vi "Load XML.vi"() -> (3 "Map":map{string, T1}(c390))   [LabVIEW 2021]
uses:
  bd.ctl
  Node/Node.lvclass
  wire.ctl
  <vilib>/xml/Load XML File.vi
  <vilib>/xml/NI_XML.lvlib
  <vilib>/httpClient/LabVIEWHTTPClient.lvlib
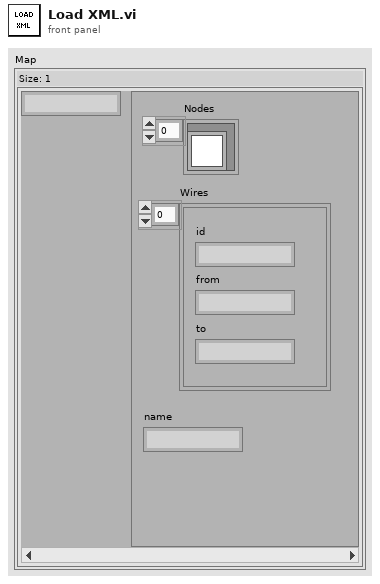
[diagram p1: front panel]
types:
  T1 = typedef "bd.ctl" = cluster{"Nodes":refnum<class "Node.lvclass">[], "Wires":T2[], "name":string}
  T2 = typedef "wire.ctl" = cluster{"id":string, "from":string, "to":string}
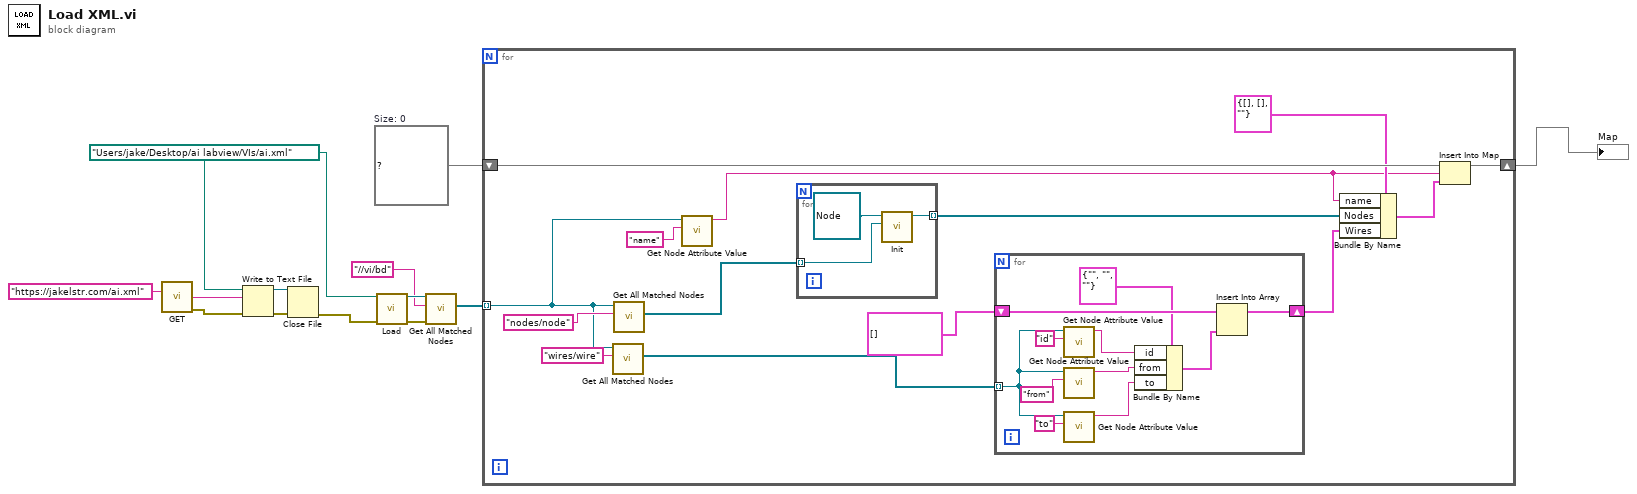
[diagram p0: block diagram]
diagram:
  w10 = map{string, T1} {}  # Size: 0
  w1 = path "/Users/jake/Desktop/ai labview/VIs/ai.xml" ("path to XML document")
  n1 = call <vilib>:"GET.vi"("url"="https://jakelstr.com/ai.xml") -> ("body"=w5:string, "error out"=w6:errorcluster)  [unwired: 11 in, 2 out]
  n2 = Write to Text File(file (use dialog)=w1, text=w5, error in=w6) -> (refnum out=w3:refnum<file>, error out=w4:errorcluster)  [unwired: 1 in, 1 out]
  n3 = Close File(refnum=w3, error in=w4) -> (error out=w2:errorcluster)  [unwired: 1 out]
  n4 = call-poly <vilib>:"Load.vi"("path to XML document"=w1, "error in (no error)"=w2) -> ("DOM document out"=w12:refnum<k20>, "error out"=w13:errorcluster)  [unwired: 11 in, 1 out]
  n5 = call <vilib>:"Get All Matched Nodes.vi"("error in (no error)"=w13, "XPath expression"="//vi/bd", "node in"=w12) -> ("node result array"=w9:refnum<k20>[])  [unwired: 6 in, 2 out]
  n6 = for {
    tunnel: w9 -> [w18] mode=indexing
    shift-right: [w26] -> w8
    shift-left: w10 -> [w27]
    n7 = call <vilib>:"Get All Matched Nodes.vi"("XPath expression"="wires/wire", "node in"=w18) -> ("node result array"=w16:refnum<k20>[])  [unwired: 7 in, 2 out]
    n8 = call <vilib>:"Get All Matched Nodes.vi"("XPath expression"="nodes/node", "node in"=w18) -> ("node result array"=w21:refnum<k20>[])  [unwired: 7 in, 2 out]
    n9 = call "Get Node Attribute Value.vi"("Attribute Name"="name", "Refnum in"=w18) -> ("Value"=w14:string)  [unwired: 9 in]
    n10 = for {
      tunnel: w21 -> [w40] mode=indexing
      tunnel: [w39] -> w20 mode=indexing
      n11 = call-dynamic "Init.vi"("Node Reg"=w40, "Node in"=refnum<class "Node.lvclass"> refnum ("Node.lvclass")) -> ("Node out"=w39:refnum<class "Node.lvclass">)  [unwired: 8 in, 1 out]
    }
    n12 = for {
      tunnel: w16 -> [w33] mode=indexing
      shift-right: [w37] -> w15
      shift-left: T2[] [] ("Wires") -> [w38]
      n13 = call "Get Node Attribute Value.vi"("Attribute Name"="id", "Refnum in"=w33) -> ("Value"=w31:string)  [unwired: 9 in]
      n14 = call "Get Node Attribute Value.vi"("Attribute Name"="from", "Refnum in"=w33) -> ("Value"=w30:string)  [unwired: 9 in]
      n15 = call "Get Node Attribute Value.vi"("Attribute Name"="to", "Refnum in"=w33) -> ("Value"=w29:string)  [unwired: 9 in]
      n16 = Bundle By Name(cluster=T2 {"id"="", "from"="", "to"=""} ("new element/subarray"), "id"=w31, "from"=w30, "to"=w29) -> (w28:T2)
      n17 = Insert Into Array(array=w38, new element=w28) -> (w37:T2[])  [unwired: 1 in]
    }
    n18 = Bundle By Name(cluster=T1 {"Nodes"=[], "Wires"=[], "name"=""} ("Block Diagram"), "name"=w14, "Nodes"=w20, "Wires"=w15) -> (w24:T1)
    n19 = Insert Into Map(map in=w27, key=w14, value=w24) -> (map out=w26:map{string, T1})  [unwired: 2 out]
  }
  "Map" <- w8
